vi "Actor Core.vi"(8 "error in":errorcluster, 11 "AE75TX in":refnum<class "AE75TX.lvclass">) -> (0 "error out":errorcluster, 3 "Actor out":refnum<class "Actor.lvclass">)   [LabVIEW 2018, in "AE75TX Actor.lvlib" / "AE75TX.lvclass"]
doc: "(<B>Filename</B>: Actor Framework.lvlib:Actor.lvclass:Actor Core.vi)\n\nReceives messages to the actor, reacts to them, and initiates any error handling that may shut the actor down.\n\nDescendant classes may override this VI to append parallel tasks for the actor to complete while it handles messages. Overrides use the Call Parent Method node."
uses:
  AE75TX.lvclass
  C:/Program Files (x86)/National Instruments/LabVIEW 2018/vi.lib/ActorFramework/Actor/Actor.lvclass
  <vilib>/ActorFramework/Actor/Actor.lvclass
  Controls/DDS State.ctl
  Controls/Modbus State.ctl
  AE75TX.lvclass/AE75TX.ctl
  <vilib>/ActorFramework/Actor/Actor.lvclass/Actor.ctl
  <vilib>/ActorFramework/Message Enqueuer/Message Enqueuer.lvclass/Message Enqueuer.ctl
  <vilib>/ORNL/CSEISMIC DDS/CSEISMIC DDS Base/CSEISMIC DDS.lvclass/CSEISMIC DDS.ctl
  <vilib>/ORNL/CSEISMIC DDS/DDS Writer/DDS Writer.lvclass
  C:/Program Files (x86)/National Instruments/LabVIEW 2018/vi.lib/ORNL/CSEISMIC DDS/CSEISMIC DDS Base/CSEISMIC DDS.lvclass
  <vilib>/ORNL/CSEISMIC DDS/DDS Reader/DDS Reader.lvclass
  <extravilib>/ChannelInstances/Stream-u16/EndpointRead.vi
  <vilib>/ActorFramework/Message Enqueuer/Init from Existing Queue.vi
  <vilib>/ActorFramework/Message Enqueuer/Enqueue.vi
  <vilib>/ORNL/CSEISMIC DDS/CSEISMIC DDS Base/Accessors/Write DDS Reference.vi
  <vilib>/ORNL/CSEISMIC DDS/CSEISMIC DDS Base/Accessors/Read DDS Reference.vi
  <extravilib>/ChannelInstances/Stream-u16/Endpoint.vi
  <vilib>/ActorFramework/Stop Msg/Stop Msg.lvclass
  C:/Program Files (x86)/National Instruments/LabVIEW 2018/vi.lib/ActorFramework/Message/Message.lvclass
  <extravilib>/ChannelInstances/Tag-t'CSEISMIC DDS.lvlib-CSEISMIC DDS.lvclass-IED_Status.ctl'/Instantiate.vi
  <extravilib>/ChannelInstances/Tag-t'CSEISMIC DDS.lvlib-CSEISMIC DDS.lvclass-DER_Status.ctl'/Instantiate.vi
  <extravilib>/ChannelInstances/Tag-t'CSEISMIC DDS.lvlib-CSEISMIC DDS.lvclass-DER_Measurement.ctl'/Instantiate.vi
  <extravilib>/ChannelInstances/Stream-u16/Instantiate.vi
  <vilib>/Modbus/master/Create Master Instance (TCP).vi
  <extravilib>/ChannelInstances/Tag-t'CSEISMIC DDS.lvlib-CSEISMIC DDS.lvclass-IED_Status.ctl'/Endpoint.vi
  <extravilib>/ChannelInstances/Tag-t'CSEISMIC DDS.lvlib-CSEISMIC DDS.lvclass-DER_Status.ctl'/Endpoint.vi
  <extravilib>/ChannelInstances/Tag-t'CSEISMIC DDS.lvlib-CSEISMIC DDS.lvclass-DER_Measurement.ctl'/Endpoint.vi
  <extravilib>/ChannelInstances/Stream-u16/)Channel.vi
  <resource>/ChannelSupport/_ChannelSupport/WaitIfNeeded.vi
  <vilib>/ActorFramework/Message Priority Queue/Priority Enqueue.vi
  <vilib>/ORNL/CSEISMIC DDS/CSEISMIC DDS Base/Error Handler.vi
  <extravilib>/ChannelInstances/Tag-t'CSEISMIC DDS.lvlib-CSEISMIC DDS.lvclass-IED_Status.ctl'/EndpointRead.vi
  <extravilib>/ChannelInstances/Tag-t'CSEISMIC DDS.lvlib-CSEISMIC DDS.lvclass-DER_Status.ctl'/EndpointRead.vi
  <extravilib>/ChannelInstances/Tag-t'CSEISMIC DDS.lvlib-CSEISMIC DDS.lvclass-DER_Measurement.ctl'/EndpointRead.vi
  <vilib>/Modbus/master/Modbus Master.lvclass
  <vilib>/ActorFramework/Message Enqueuer/Message Enqueuer.lvclass
  <vilib>/RTI DDS Toolkit/Library/LVDDS_library.lvlib
  <extravilib>/ChannelInstances/Tag-t'CSEISMIC DDS.lvlib-CSEISMIC DDS.lvclass-IED_Status.ctl'.lvlib
  <extravilib>/ChannelInstances/Tag-t'CSEISMIC DDS.lvlib-CSEISMIC DDS.lvclass-DER_Status.ctl'.lvlib
  <extravilib>/ChannelInstances/Tag-t'CSEISMIC DDS.lvlib-CSEISMIC DDS.lvclass-DER_Measurement.ctl'.lvlib
  <extravilib>/ChannelInstances/Stream-u16.lvlib
panel:
  out "MicrogridID":u8
  out "DDS State":T1
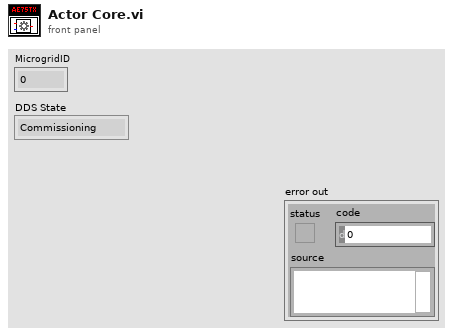
[diagram p1: front panel]
types:
  T1 = typedef "AE75TX Actor.lvlib/AE75TX.lvclass/DDS State.ctl" = enum16{"Commissioning", "CheckID", "InitDDS", "ReadDDS", "WriteDDS", "CheckClose", "Close", "Shutdown"}
  T2 = typedef "AE75TX Actor.lvlib/AE75TX.lvclass/Modbus State.ctl" = enum16{"Initialize", "Read", "Write", "Close"}
  T3 = typedef "AE75TX Actor.lvlib/AE75TX.lvclass/Scaling Coefficients Measurements.ctl" = cluster{"Current":dbl, "Voltage":dbl, "Real Power":dbl, "Reactive Power":dbl, "Frequency":dbl}
  T4 = typedef "AE75TX Actor.lvlib/AE75TX.lvclass/Modbus Configuration Cluster.ctl" = cluster{"IP Address":string, "Port":u16, "DeviceID":T5}
  T5 = typedef "CSEISMIC DDS.lvlib/CSEISMIC DDS.lvclass/DeviceID.ctl" = string
  T6 = typedef "CSEISMIC DDS.lvlib/CSEISMIC DDS.lvclass/DER_Info.ctl" = cluster{"DeviceID":T5, "LineConfig":u8[], "NominalVoltage(V)":dbl, "PowerRating(kVA)":dbl, "VFControl":bool, "PControl":bool, "QControl":bool, "PFControl":bool, "PVControl":bool, "Droop":bool, "DroopConfigurable":bool, "Unbalanced":bool}
  T7 = typedef "CSEISMIC DDS.lvlib/CSEISMIC DDS.lvclass/DER_Measurement.ctl" = cluster{"DeviceID":T5, "Voltage":dbl[], "Current":dbl[], "RealPower":dbl[], "ReactivePower":dbl[], "LineConfig":u8[], "Frequency":dbl}
  T8 = typedef "CSEISMIC DDS.lvlib/CSEISMIC DDS.lvclass/DER_Status.ctl" = cluster{"DeviceID":T5, "VFControl":bool, "PControl":bool, "QControl":bool, "PFControl":bool, "PVControl":bool, "Droop":bool, "Unbalanced":bool, "MicrogridVF":bool, "RealDroop(kW)":T9, "ReactiveDroop(kVar)":T9}
  T9 = typedef "CSEISMIC DDS.lvlib/CSEISMIC DDS.lvclass/DroopCurve.ctl" = cluster{"XMin":dbl, "XMax":dbl, "YMin":dbl, "YMax":dbl}
  T10 = typedef "CSEISMIC DDS.lvlib/CSEISMIC DDS.lvclass/IED_Status.ctl" = cluster{"DeviceID":T5, "Timestamp":T11, "MicrogridID":u8, "Active":bool, "Inactive":bool, "Error":i32, "Fault":bool, "ErrorString":string}
  T11 = typedef "CSEISMIC DDS.lvlib/CSEISMIC DDS.lvclass/Timestamp.ctl" = cluster{"Seconds":u64, "Remainder":u64}
  T12 = typedef "Tag-t'CSEISMIC DDS.lvlib-CSEISMIC DDS.lvclass-DER_Status.ctl'.lvlib/))Channel.ctl" = refnum<queue>
  T13 = typedef "Tag-t'CSEISMIC DDS.lvlib-CSEISMIC DDS.lvclass-DER_Measurement.ctl'.lvlib/))Channel.ctl" = refnum<queue>
  T14 = typedef "Tag-t'CSEISMIC DDS.lvlib-CSEISMIC DDS.lvclass-IED_Status.ctl'.lvlib/))Channel.ctl" = refnum<queue>
  T15 = typedef "CSEISMIC DDS.lvlib/CSEISMIC DDS.lvclass/IED_setMicrogridID.ctl" = cluster{"DeviceID":T5, "MicrogridID":u8}
  T16 = typedef "LVDDS_library.lvlib/DDS Sample Info.ctl" = cluster{"DDS_SampleStateKind":enum32{"DDS_INVALID_SAMPLE_STATE", "DDS_READ_SAMPLE_STATE", "DDS_NOT_READ_SAMPLE_STATE"}, "DDS_ViewStateKind":enum32{"DDS_INVALID_SAMPLE_STATE", "DDS_NEW_VIEW_STATE", "DDS_NOT_NEW_VIEW_STATE"}, "DDS_InstanceStateKind":enum32{"DDS_INVALID_STATE", "DDS_ALIVE_INSTANCE_STATE", "DDS_NOT_ALIVE_DISPOSED_INSTANCE_STATE", "", "DDS_NOT_ALIVE_NO_WRITERS_INSTANCE_STATE"}, "sec":i32, "nanosec":u32, "valid_data":bool}
  T17 = typedef "CSEISMIC DDS.lvlib/CSEISMIC DDS.lvclass/DER_SetPointP.ctl" = cluster{"DeviceID":T5, "RealPower (kW)":dbl[]}
  T18 = typedef "Stream-u16.lvlib/)Channel.ctl" = refnum<queue>
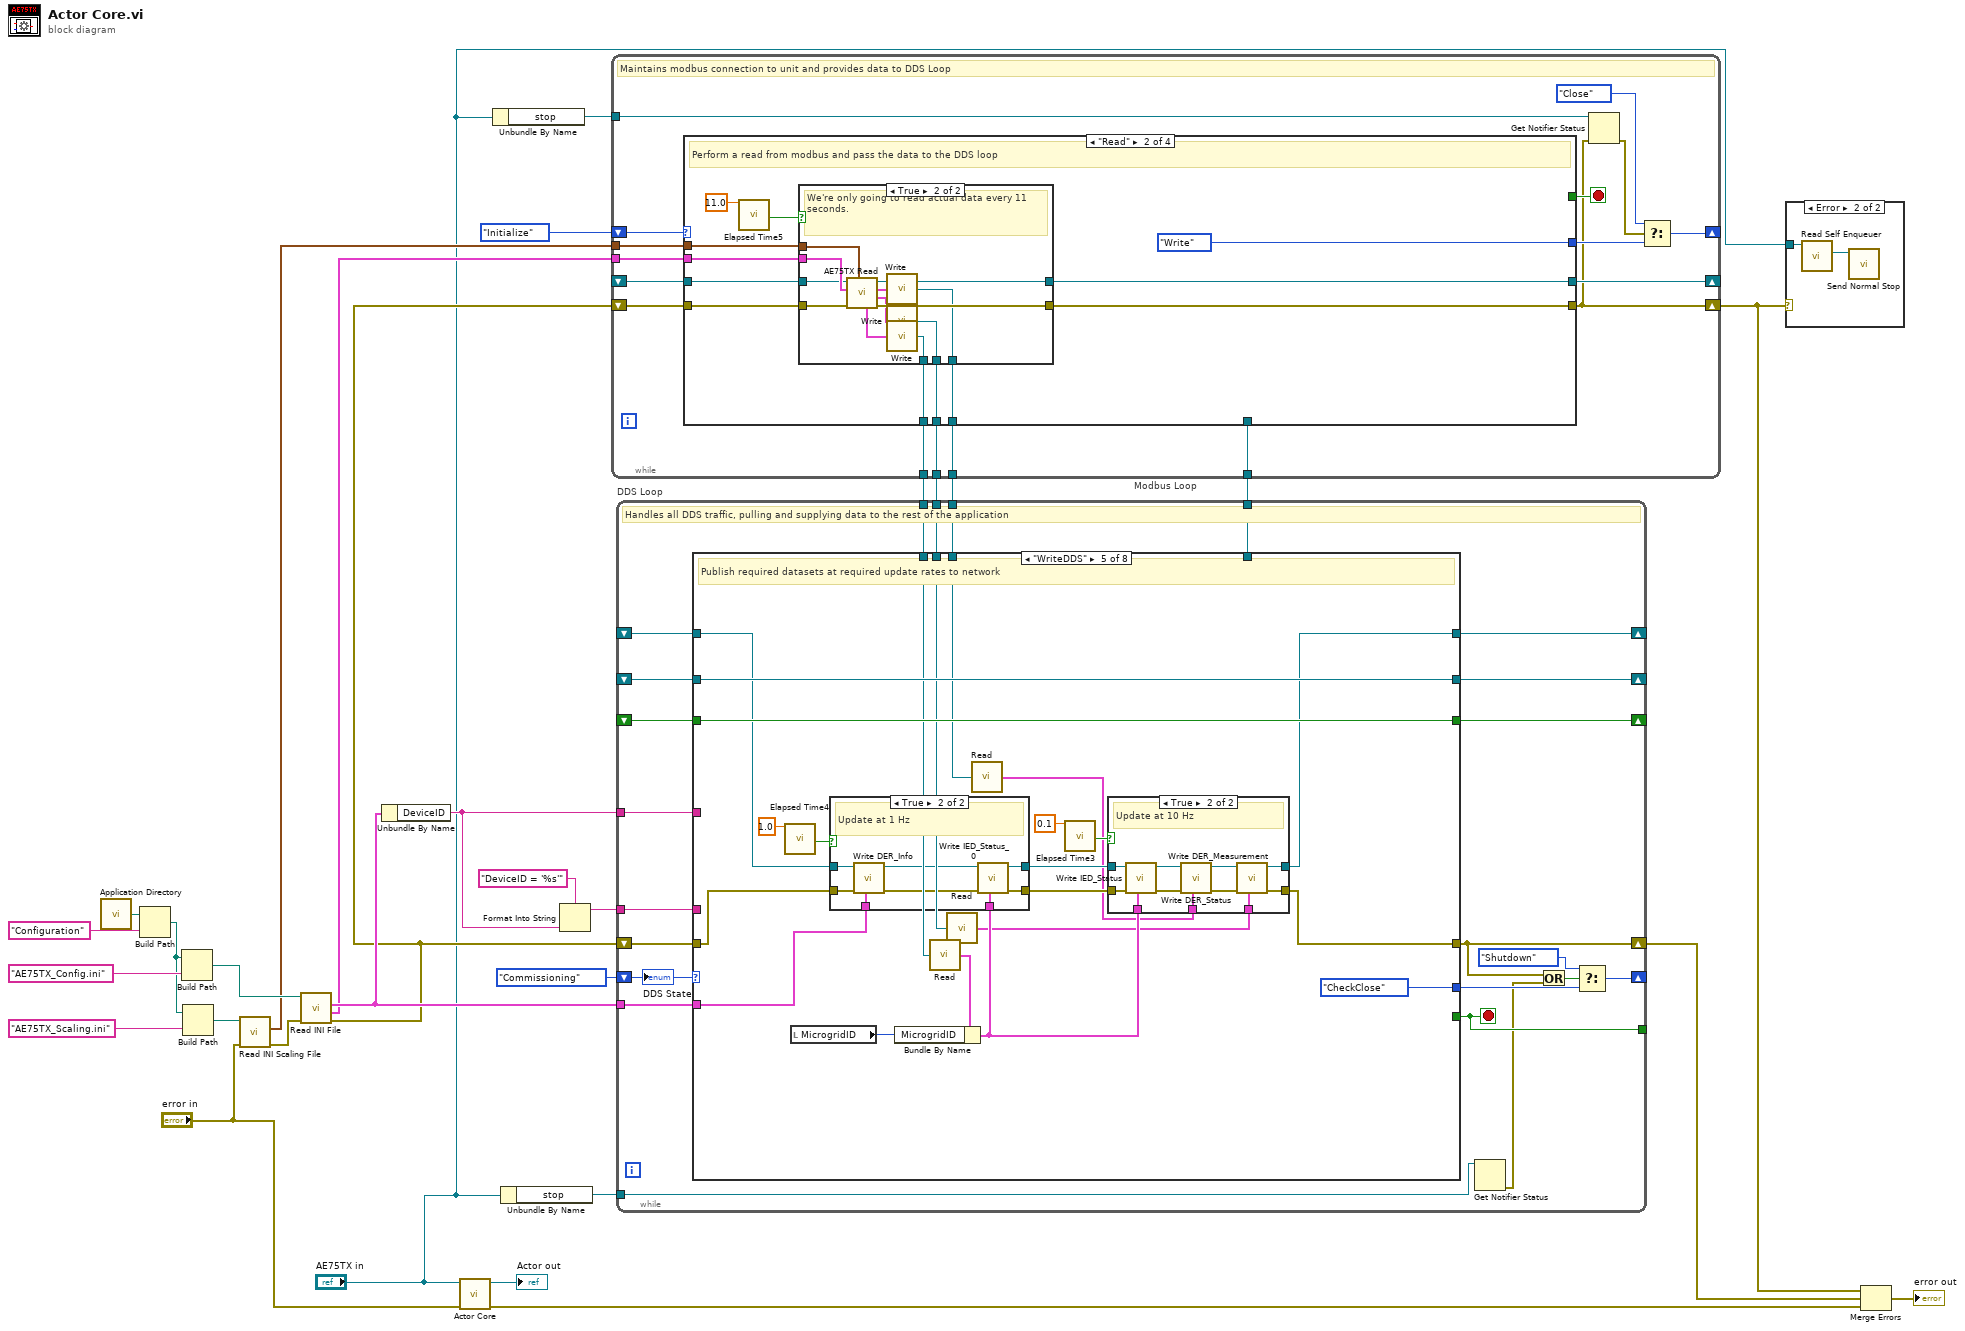
[diagram p0: block diagram]
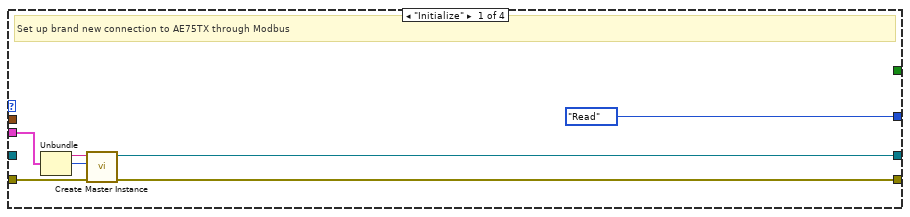
[diagram p3: hidden frame]
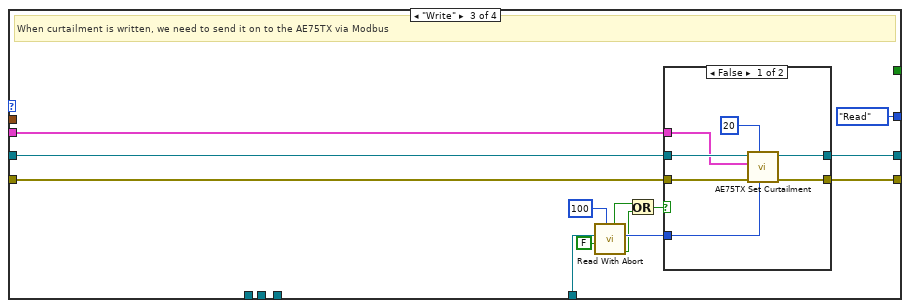
[diagram p5: hidden frame]
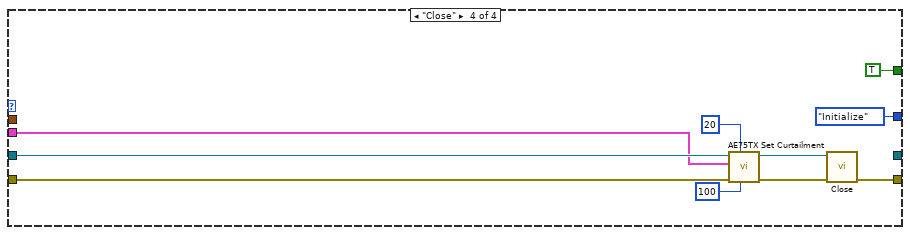
[diagram p7: hidden frame]
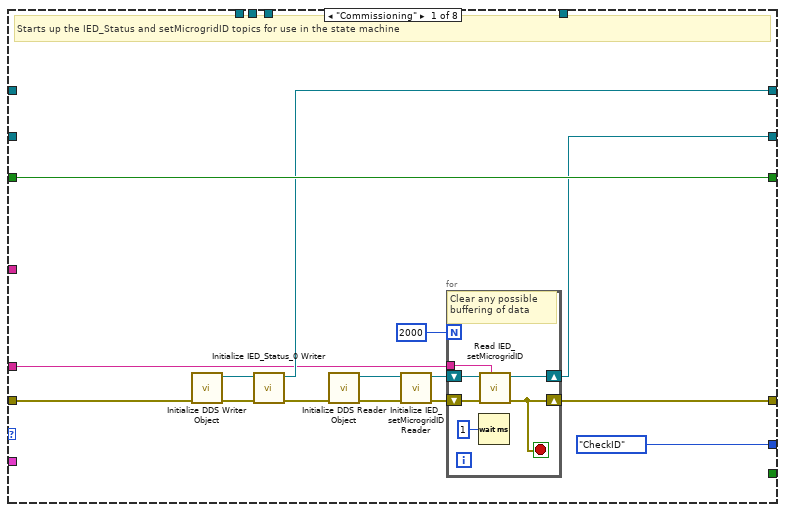
[diagram p8: hidden frame]
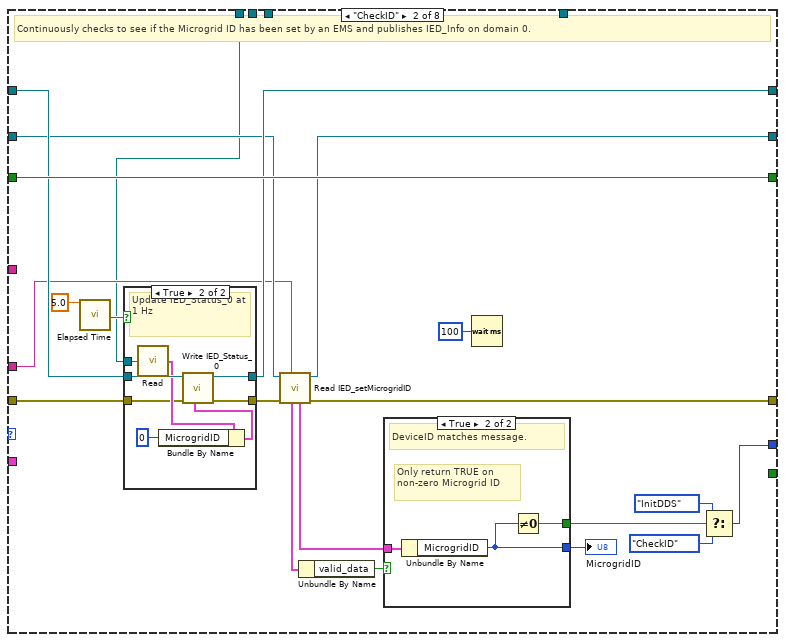
[diagram p9: hidden frame]
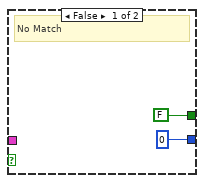
[diagram p11: hidden frame]
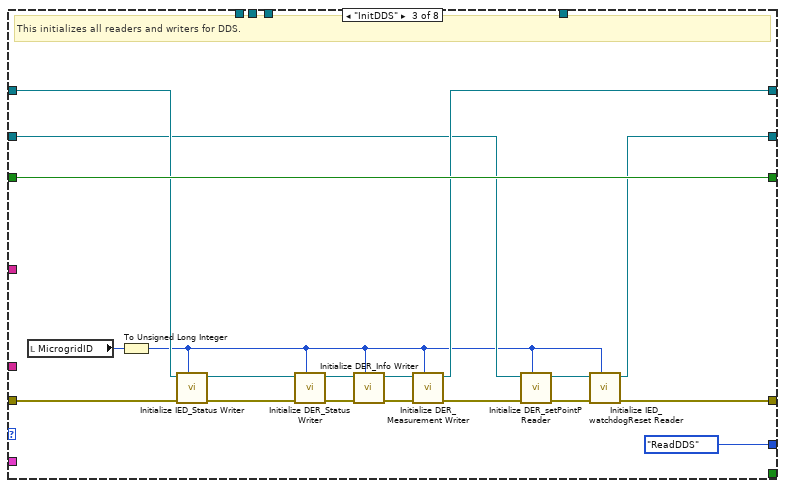
[diagram p12: hidden frame]
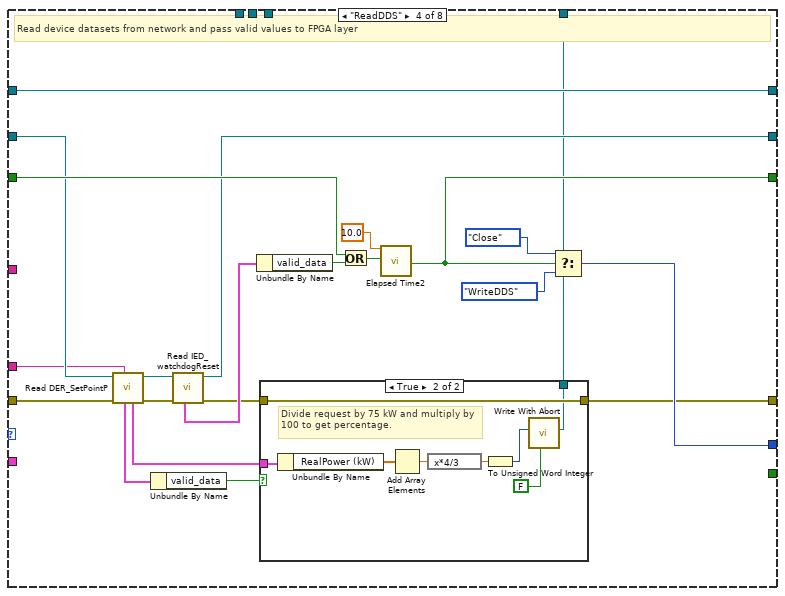
[diagram p13: hidden frame]
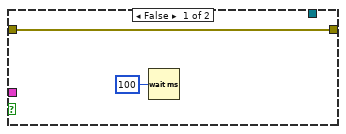
[diagram p14: hidden frame]
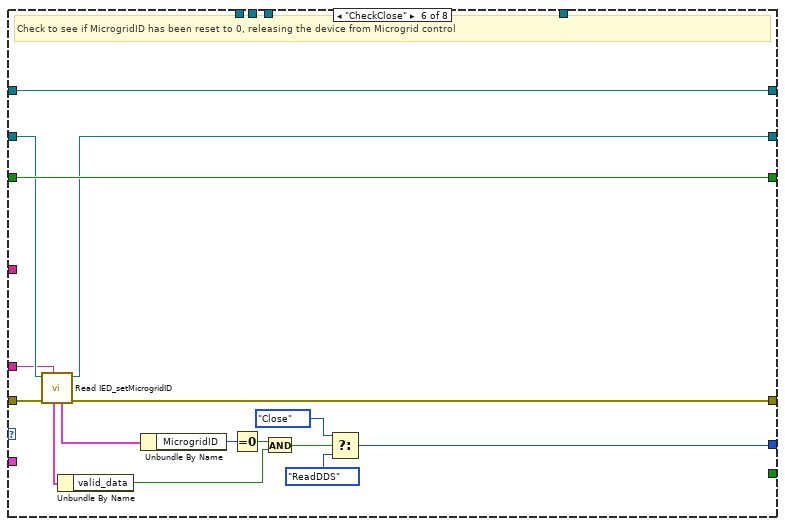
[diagram p17: hidden frame]
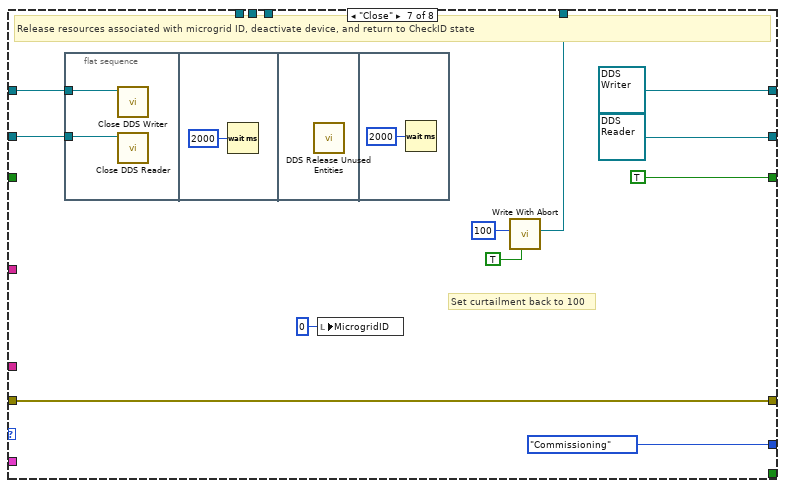
[diagram p18: hidden frame]
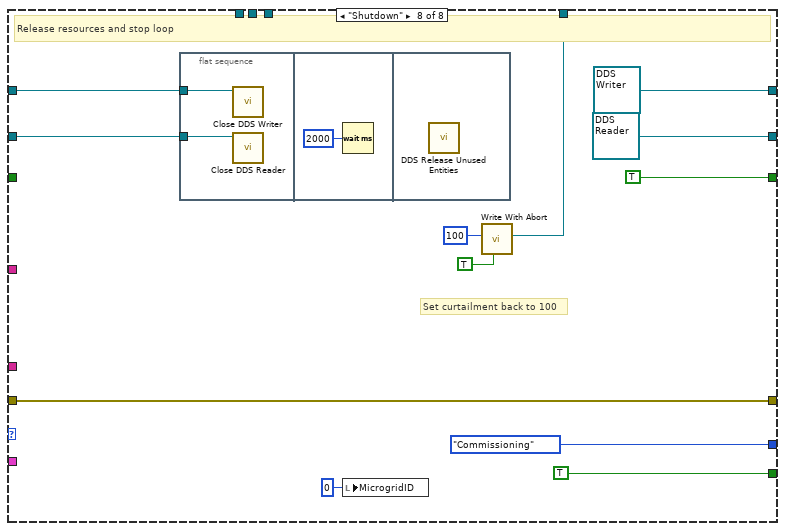
[diagram p19: hidden frame]
diagram:
  n1 = call <vilib>:"Application Directory.vi"() -> ("Application Directory"=w25:path)
  n2 = Build Path(base path=w25, name or relative path="Configuration") -> (appended path=w17:path)
  n3 = Build Path(base path=w17, name or relative path="AE75TX_Config.ini") -> (appended path=w20:path)
  n4 = Build Path(base path=w17, name or relative path="AE75TX_Scaling.ini") -> (appended path=w16:path)
  n5 = call "Read INI Scaling File.vi"("error in"="error in", "Path"=w16) -> ("error out"=w19:errorcluster, "Scaling Coefficients"=w7:T3)  [unwired: 8 in]
  n6 = call "Read INI File.vi"("error in"=w19, "Path"=w20) -> ("error out"=w8:errorcluster, "Modbus Configuration"=w9:T4, "DER_Info"=w12:T6)  [unwired: 7 in]
  n7 = Unbundle By Name(w12) -> ("DeviceID"=w23:T5)
  n8 = call-parent "Actor Core.vi"("error in"="error in", "Actor in"="AE75TX in") -> ("error out"=w30:errorcluster, "Actor out"=→"Actor out":refnum<class "Actor.lvclass">)  [unwired: 8 in]
  n9 = Unbundle By Name("AE75TX in") -> ("stop"=w11:refnum<notifier>)
  n10 = Unbundle By Name("AE75TX in") -> ("stop"=w14:refnum<notifier>)
  n11 = Format Into String(format string="DeviceID = '%s'" ("Query condition"), w23) -> (resulting string=w22:string)  [unwired: 2 in, 1 out]
  n12 = while "Modbus Loop" {
    tunnel: w11 -> [w47]
    shift-right: [w33] -> _
    shift-left: Modbus_State."Initialize" -> [w46]
    tunnel: w9 -> [w45]
    shift-right: [w44] -> _
    shift-left: _ -> [w42]
    shift-right: [w31] -> w1
    shift-left: w8 -> [w43]
    tunnel: w7 -> [w41]
    tunnel: w6 -> [w40]
    tunnel: [w39] -> w5
    tunnel: [w38] -> w4
    tunnel: [w37] -> w3
    stop <- w36 stop-if-true
    # "Maintains modbus connection to unit and provides data to DDS Loop"
    n13 = case shown="\"Read\"" w46 {
      tunnel: w45 -> [w52 w66 w87 w104]
      tunnel: [w51 w63 w85 _] -> w44
      tunnel: w43 -> [w50 w64 w92 w106]
      tunnel: [w49 w62 w84 w112] -> w31
      tunnel: [Modbus_State."Read" Modbus_State."Write" Modbus_State."Read" Modbus_State."Initialize"] -> w34
      tunnel: w42 -> [_ w65 w93 w107]
      tunnel: w41 -> [_ w58 _ _]
      tunnel: w40 -> [_ _ w91 _]
      tunnel: [_ w57 _ _] -> w39
      tunnel: [_ w56 _ _] -> w38
      tunnel: [_ w55 _ _] -> w37
      tunnel: [_ _ _ TRUE] -> w36
      frame "Initialize" {
        # "Set up brand new connection to AE75TX through Modbus"
        n14 = Unbundle(w52) -> ("IP Address"=w53:string, "Port"=w54:u16)  [unwired: 1 out]
        n15 = call-poly <vilib>:"Create Master Instance.vi"("error in (no error)"=w50, "port (502)"=w54, "address"=w53) -> ("error out"=w49:errorcluster, "TCP master instance"=w51:refnum<class "Modbus Master.lvclass">)  [unwired: 7 in]
      }
      frame "Read" {
        # "Perform a read from modbus and pass the data to the DDS loop"
        n16 = call "Elapsed Time5"("Time Target (s)"=11.0) -> ("Time has Elapsed"=w60:bool)  [unwired: 11 in, 7 out]
        n17 = case shown="True" w60 {
          tunnel: w66 -> [_ w80]
          tunnel: w65 -> [w67 w79]
          tunnel: w64 -> [w68 w78]
          tunnel: [w67 w77] -> w63
          tunnel: [w68 w76] -> w62
          tunnel: w58 -> [_ w75]
          tunnel: [_ w72] -> w57
          tunnel: [_ w71] -> w56
          tunnel: [_ w70] -> w55
          frame False {
            # "Do nothing"
          }
          frame True {
            # "We're only going to read actual data every 11 seconds."
            n18 = call "AE75TX Read.vi"("Scaling Coefficients"=w75, "error in"=w78, "Modbus Configuration"=w80, "Modbus Master in"=w79) -> ("error out"=w76:errorcluster, "DER_Measurement"=w73:T7, "DER_Status"=w74:T8, "Modbus Master out"=w77:refnum<class "Modbus Master.lvclass">, "IED_Status"=w69:T10)  [unwired: 3 in]
            n19 = call <extravilib>:"Write.vi"("element"=w74) -> ("channel"=w71:T12)  [unwired: 1 out]
            n20 = call <extravilib>:"Write.vi"("element"=w73) -> ("channel"=w72:T13)  [unwired: 1 out]
            n21 = call <extravilib>:"Write.vi"("element"=w69) -> ("channel"=w70:T14)  [unwired: 1 out]
          }
        }
      }
      frame "Write" {
        # "When curtailment is written, we need to send it on to the AE75TX via Modbus"
        n22 = call <extravilib>:"Read With Abort.vi"("timeout in ms (-1)"=100, "abort"=FALSE, "channel"=w91) -> ("element"=w90:u16, "aborted?"=w81:bool, "timed out?"=w88:bool)  [unwired: 3 in, 3 out]
        n23 = Or(x=w88, y=w81) -> (x .or. y?=w82:bool)
        n24 = case shown="False" w82 {
          tunnel: w93 -> [w99 w102]
          tunnel: w92 -> [w98 w101]
          tunnel: w90 -> [w94 _]
          tunnel: [w97 w102] -> w85
          tunnel: [w96 w101] -> w84
          tunnel: w87 -> [w95 _]
          frame False {
            n25 = call "AE75TX Set Curtailment.vi"("Curtailment (%)"=w94, "Ramp Rate (kVA/s)"=u16 20, "error in"=w98, "Modbus Configuration"=w95, "Modbus Master in"=w99) -> ("error out"=w96:errorcluster, "Modbus Master out"=w97:refnum<class "Modbus Master.lvclass">)  [unwired: 5 in]
          }
          frame True {
          }
        }
      }
      frame "Close" {
        n26 = call "AE75TX Set Curtailment.vi"("Curtailment (%)"=u16 100, "Ramp Rate (kVA/s)"=u16 20, "error in"=w106, "Modbus Configuration"=w104, "Modbus Master in"=w107) -> ("error out"=w108:errorcluster, "Modbus Master out"=w109:refnum<class "Modbus Master.lvclass">)  [unwired: 5 in]
        n27 = call-dynamic "Close.vi"("error in (no error)"=w108, "Modbus master in"=w109) -> ("error out"=w112:errorcluster)  [unwired: 9 in]
      }
    }
    n28 = Get Notifier Status(notifier=w47, error in (no error)=w31) -> (error out=w35:errorcluster)  [unwired: 4 out]
    n29 = Select(t=Modbus_State."Close", s=w35, f=w34) -> (s? t:f=w33:T2)
  }
  n30 = while "DDS Loop" {
    shift-right: [w133] -> _
    shift-left: DDS_State."Commissioning" -> [w135]
    tunnel: w23 -> [w134]
    shift-right: [w121] -> w13
    shift-left: w8 -> [w117]
    shift-right: [w122] -> _
    shift-left: _ -> [w129]
    tunnel: [w128] -> _
    tunnel: w22 -> [w123]
    shift-right: [w125] -> _
    shift-left: _ -> [w127]
    shift-right: [w124] -> _
    shift-left: _ -> [w126]
    tunnel: w12 -> [w120]
    tunnel: w14 -> [w119]
    tunnel: [w116] -> w6
    tunnel: w5 -> [w114]
    tunnel: w4 -> [w113]
    tunnel: w3 -> [w115]
    stop <- w128 stop-if-true
    # "Handles all DDS traffic, pulling and supplying data to the rest of the application"
    n31 = case shown="\"CheckID\"" w135 {
      tunnel: [DDS_State."CheckID" w173 DDS_State."ReadDDS" w231 DDS_State."CheckClose" w301 DDS_State."Commissioning" ("f") DDS_State."Commissioning" ("f")] -> w132
      tunnel: [w149 w166 w206 w220 w262 w297 w314 w323] -> w121
      tunnel: w134 -> [_ _ _ _ _ _ _ _]
      tunnel: w117 -> [w136 w157 w208 w218 w244 w298 w314 w323]
      tunnel: [_ _ _ _ _ _ _ TRUE] -> w128
      tunnel: [w148 w169 w209 w228 w257 w300 TRUE ("Time has Elapsed") TRUE ("Time has Elapsed")] -> w122
      tunnel: w129 -> [w148 w169 w209 w227 w257 w300 _ _]
      tunnel: w127 -> [_ w168 w205 w226 w255 w293 w311 w325]
      tunnel: w126 -> [_ w164 w197 w219 w256 w299 w310 w324]
      tunnel: [w146 w167 w203 w226 w254 w293 refnum<class "DDS Writer.lvclass"> refnum ("DDS Writer out") refnum<class "DDS Writer.lvclass"> refnum ("DDS Writer out")] -> w125
      tunnel: [w145 w163 w202 w222 w256 w294 refnum<class "DDS Reader.lvclass"> refnum ("DDS Reader out") refnum<class "DDS Reader.lvclass"> refnum ("DDS Reader out")] -> w124
      tunnel: w123 -> [w138 w161 _ w213 _ w295 _ _]
      tunnel: w120 -> [_ _ _ _ w253 _ _ _]
      tunnel: [_ _ _ w212 _ _ w307 w320] -> w116
      tunnel: w115 -> [_ w158 _ _ w250 _ _ _]
      tunnel: w114 -> [_ _ _ _ w249 _ _ _]
      tunnel: w113 -> [_ _ _ _ w248 _ _ _]
      frame "Commissioning" {
        # "Starts up the IED_Status and setMicrogridID topics for use in the state machine"
        n32 = call <vilib>:"Initialize DDS Writer Object.vi"("error in"=w136) -> ("error out"=w143:errorcluster, "DDS Writer out"=w142:refnum<class "DDS Writer.lvclass">)  [unwired: 9 in]
        n33 = call <vilib>:"Initialize IED_Status_0 Writer.vi"("error in"=w143, "DDS Writer in"=w142) -> ("error out"=w141:errorcluster, "DDS Writer out"=w146:refnum<class "DDS Writer.lvclass">)  [unwired: 8 in]
        n34 = call <vilib>:"Initialize DDS Reader Object.vi"("error in"=w141) -> ("error out"=w140:errorcluster, "DDS Reader out"=w139:refnum<class "DDS Reader.lvclass">)  [unwired: 9 in]
        n35 = call <vilib>:"Initialize IED_setMicrogridID Reader.vi"("error in"=w140, "DDS Reader in"=w139) -> ("error out"=w144:errorcluster, "DDS Reader out"=w147:refnum<class "DDS Reader.lvclass">)  [unwired: 8 in]
        n36 = for {
          N: 2000 -> [_]
          shift-right: [w154] -> w145
          shift-left: w147 -> [w155]
          shift-right: [w152] -> w149
          shift-left: w144 -> [w153]
          tunnel: w138 -> [w151]
          stop <- w152 stop-if-true
          # "Clear any possible buffering of data"
          n37 = Wait (ms)(milliseconds to wait=u32 1) -> ()  [unwired: 1 out]
          n38 = call <vilib>:"Read IED_setMicrogridID.vi"("Query condition"=w151, "error in"=w153, "DDS Reader in"=w155) -> ("error out"=w152:errorcluster, "DDS Reader out"=w154:refnum<class "DDS Reader.lvclass">)  [unwired: 5 in, 2 out]
        }
      }
      frame "CheckID" {
        # "Continuously checks to see if the Microgrid ID has been set by an EMS and publishes IED_Info on domain 0."
        n39 = call "Elapsed Time"("Time Target (s)"=5.0) -> ("Time has Elapsed"=w171:bool)  [unwired: 11 in, 7 out]
        n40 = case shown="True" w171 {
          tunnel: [w178 w186] -> w165
          tunnel: w168 -> [w179 w187]
          tunnel: [w179 w185] -> w167
          tunnel: w158 -> [_ w183]
          tunnel: w157 -> [w178 w180]
          frame False {
          }
          frame True {
            # "Update IED_Status_0 at 1 Hz"
            n41 = call <extravilib>:"Read.vi"("channel"=w183) -> ("element"=w182:T10)  [unwired: 1 in, 1 out]
            n42 = Bundle By Name(cluster=w182, "MicrogridID"=u8 0) -> (w181:T10)
            n43 = call <vilib>:"Write IED_Status_0.vi"("IED_Status"=w181, "error in"=w180, "DDS Writer in"=w187) -> ("error out"=w186:errorcluster, "DDS Writer out"=w185:refnum<class "DDS Writer.lvclass">)  [unwired: 7 in]
          }
        }
        n44 = call <vilib>:"Read IED_setMicrogridID.vi"("Query condition"=w161, "error in"=w165, "DDS Reader in"=w164) -> ("error out"=w166:errorcluster, "DDS Reader out"=w163:refnum<class "DDS Reader.lvclass">, "data"=w162:T15, "DDS Sample Info"=w160:T16)  [unwired: 5 in]
        n45 = Unbundle By Name(w160) -> ("valid_data"=w159:bool)
        n46 = case shown="True" w159 {
          tunnel: w162 -> [_ w192]
          tunnel: [u8 0 ("MicrogridID") w191] -> w172
          tunnel: [FALSE w190] -> w176
          frame False {
            # "No Match"
          }
          frame True {
            # "Only return TRUE on non-zero Microgrid ID"
            # "DeviceID matches message."
            n47 = Unbundle By Name(w192) -> ("MicrogridID"=w191:u8)
            n48 = Not Equal To 0?(x=w191) -> (x != 0?=w190:bool)
          }
        }
        "MicrogridID" <- w172
        n49 = Wait (ms)(milliseconds to wait=u32 100) -> ()  [unwired: 1 out]
        n50 = Select(t=DDS_State."InitDDS", s=w176, f=DDS_State."CheckID") -> (s? t:f=w173:T1)
      }
      frame "InitDDS" {
        # "This initializes all readers and writers for DDS."
        n51 = local read "MicrogridID"() -> (w210:u8)
        n52 = To Unsigned Long Integer(number=w210) -> (unsigned 32bit integer=w193:u32)
        n53 = call <vilib>:"Initialize IED_Status Writer.vi"("MicrogridID"=w193, "error in"=w208, "DDS Writer in"=w205) -> ("error out"=w200:errorcluster, "DDS Writer out"=w201:refnum<class "DDS Writer.lvclass">)  [unwired: 7 in]
        n54 = call <vilib>:"Initialize DER_Status Writer.vi"("MicrogridID"=w193, "error in"=w200, "DDS Writer in"=w201) -> ("error out"=w199:errorcluster, "DDS Writer out"=w198:refnum<class "DDS Writer.lvclass">)  [unwired: 7 in]
        n55 = call <vilib>:"Initialize DER_Info Writer.vi"("MicrogridID"=w193, "error in"=w199, "DDS Writer in"=w198) -> ("error out"=w207:errorcluster, "DDS Writer out"=w204:refnum<class "DDS Writer.lvclass">)  [unwired: 7 in]
        n56 = call <vilib>:"Initialize DER_Measurement Writer.vi"("MicrogridID"=w193, "error in"=w207, "DDS Writer in"=w204) -> ("error out"=w196:errorcluster, "DDS Writer"=w203:refnum<class "DDS Writer.lvclass">)  [unwired: 7 in]
        n57 = call <vilib>:"Initialize DER_setPointP Reader.vi"("MicrogridID"=w193, "error in"=w196, "DDS Reader in"=w197) -> ("error out"=w194:errorcluster, "DDS Reader out"=w195:refnum<class "DDS Reader.lvclass">)  [unwired: 7 in]
        n58 = call <vilib>:"Initialize IED_watchdogReset Reader.vi"("MicrogridID"=w193, "error in"=w194, "DDS Reader in"=w195) -> ("error out"=w206:errorcluster, "DDS Reader out"=w202:refnum<class "DDS Reader.lvclass">)  [unwired: 7 in]
      }
      frame "ReadDDS" {
        # "Read device datasets from network and pass valid values to FPGA layer"
        n59 = call <vilib>:"Read DER_SetPointP.vi"("Query condition"=w213, "error in"=w218, "DDS Reader in"=w219) -> ("error out"=w216:errorcluster, "DDS Reader out"=w217:refnum<class "DDS Reader.lvclass">, "data"=w214:T17, "DDS Sample Info"=w215:T16)  [unwired: 5 in]
        n60 = Unbundle By Name(w215) -> ("valid_data"=w223:bool)
        n61 = call <vilib>:"Read IED_watchdogReset.vi"("error in"=w216, "DDS Reader in"=w217) -> ("error out"=w221:errorcluster, "DDS Reader out"=w222:refnum<class "DDS Reader.lvclass">, "DDS Sample Info"=w225:T16)  [unwired: 6 in, 1 out]
        n62 = Unbundle By Name(w225) -> ("valid_data"=w224:bool)
        n63 = case shown="True" w223 {
          tunnel: w221 -> [w235 w238]
          tunnel: [w235 w238] -> w220
          tunnel: w214 -> [_ w243]
          tunnel: [_ w237] -> w212
          frame False {
            n64 = Wait (ms)(milliseconds to wait=u32 100) -> ()  [unwired: 1 out]
          }
          frame True {
            # "Divide request by 75 kW and multiply by 100 to get percentage."
            n65 = Unbundle By Name(w243) -> ("RealPower (kW)"=w242:dbl[])
            n66 = Add Array Elements(numeric array=w242) -> (sum=w241:dbl)
            n67 = expression code="x*4/3"(w241) -> (w240:dbl)
            n68 = To Unsigned Word Integer(number=w240) -> (unsigned 16bit integer=w239:u16)
            n69 = call <extravilib>:"Write With Abort.vi"("abort"=FALSE, "element"=w239) -> ("channel"=w237:T18)  [unwired: 6 in, 3 out]
          }
        }
        n70 = Or(x=w227, y=w224) -> (x .or. y?=w229:bool)
        n71 = call "Elapsed Time2"("Time Target (s)"=10.0, "Reset"=w229) -> ("Time has Elapsed"=w228:bool)  [unwired: 10 in, 7 out]
        n72 = Select(t=DDS_State."Close", s=w228, f=DDS_State."WriteDDS") -> (s? t:f=w231:T1)
      }
      frame "WriteDDS" {
        # "Publish required datasets at required update rates to network"
        n73 = call "Elapsed Time4"("Time Target (s)"=1.0) -> ("Time has Elapsed"=w258:bool)  [unwired: 11 in, 7 out]
        n74 = local read "MicrogridID"() -> (w251:u8)
        n75 = call <extravilib>:"Read.vi"("channel"=w250) -> ("element"=w247:T10)  [unwired: 1 in, 1 out]
        n76 = Bundle By Name(cluster=w247, "MicrogridID"=w251) -> (w252:T10)
        n77 = case shown="True" w258 {
          tunnel: [w280 w287] -> w264
          tunnel: [w279 w288] -> w263
          tunnel: w253 -> [_ w286]
          tunnel: w255 -> [w280 w285]
          tunnel: w252 -> [_ w282]
          tunnel: w244 -> [w279 w281]
          frame False {
          }
          frame True {
            # "Update at 1 Hz"
            n78 = call <vilib>:"Write DER_Info.vi"("DER_Info"=w286, "error in"=w281, "DDS Writer in"=w285) -> ("error out"=w284:errorcluster, "DDS Writer out"=w283:refnum<class "DDS Writer.lvclass">)  [unwired: 7 in]
            n79 = call <vilib>:"Write IED_Status_0.vi"("IED_Status"=w282, "error in"=w284, "DDS Writer in"=w283) -> ("error out"=w288:errorcluster, "DDS Writer out"=w287:refnum<class "DDS Writer.lvclass">)  [unwired: 7 in]
          }
        }
        n80 = call <extravilib>:"Read.vi"("channel"=w249) -> ("element"=w245:T7)  [unwired: 1 in, 1 out]
        n81 = call <extravilib>:"Read.vi"("channel"=w248) -> ("element"=w246:T8)  [unwired: 1 in, 1 out]
        n82 = call "Elapsed Time3"("Time Target (s)"=0.1) -> ("Time has Elapsed"=w260:bool)  [unwired: 11 in, 7 out]
        n83 = case shown="True" w260 {
          tunnel: w264 -> [w267 w278]
          tunnel: w263 -> [w266 w277]
          tunnel: [w267 w276] -> w254
          tunnel: [w266 w275] -> w262
          tunnel: w252 -> [_ w268]
          tunnel: w246 -> [_ w270]
          tunnel: w245 -> [_ w269]
          frame False {
          }
          frame True {
            # "Update at 10 Hz"
            n84 = call <vilib>:"Write IED_Status.vi"("IED_Status"=w268, "error in"=w277, "DDS Writer in"=w278) -> ("error out"=w274:errorcluster, "DDS Writer out"=w273:refnum<class "DDS Writer.lvclass">)  [unwired: 7 in]
            n85 = call <vilib>:"Write DER_Status.vi"("DER_Status"=w270, "error in"=w274, "DDS Writer in"=w273) -> ("error out"=w272:errorcluster, "DDS Writer out"=w271:refnum<class "DDS Writer.lvclass">)  [unwired: 7 in]
            n86 = call <vilib>:"Write DER_Measurement.vi"("DER_Measurement"=w269, "error in"=w272, "DDS Writer in"=w271) -> ("error out"=w275:errorcluster, "DDS Writer out"=w276:refnum<class "DDS Writer.lvclass">)  [unwired: 7 in]
          }
        }
      }
      frame "CheckClose" {
        # "Check to see if MicrogridID has been reset to 0, releasing the device from Microgrid control"
        n87 = call <vilib>:"Read IED_setMicrogridID.vi"("Query condition"=w295, "error in"=w298, "DDS Reader in"=w299) -> ("error out"=w297:errorcluster, "DDS Reader out"=w294:refnum<class "DDS Reader.lvclass">, "data"=w296:T15, "DDS Sample Info"=w292:T16)  [unwired: 5 in]
        n88 = Unbundle By Name(w292) -> ("valid_data"=w291:bool)
        n89 = Unbundle By Name(w296) -> ("MicrogridID"=w304:u8)
        n90 = Equal To 0?(x=w304) -> (x = 0?=w290:bool)
        n91 = And(x=w290, y=w291) -> (x .and. y?=w289:bool)
        n92 = Select(t=DDS_State."Close", s=w289, f=DDS_State."ReadDDS") -> (s? t:f=w301:T1)
      }
      frame "Close" {
        # "Set curtailment back to 100"
        # "Release resources associated with microgrid ID, deactivate device, and return to CheckID state"
        n93 = flat-sequence {
          tunnel: w311 -> [w317]
          tunnel: w310 -> [w316]
          frame #0 {
            n94 = call <vilib>:"Close DDS Writer.vi"("DDS Writer in"=w317) -> ()  [unwired: 10 in, 1 out]
            n95 = call <vilib>:"Close DDS Reader.vi"("DDS Reader in"=w316) -> ()  [unwired: 10 in, 1 out]
          }
          frame #1 {
            n96 = Wait (ms)(milliseconds to wait=u32 2000) -> ()  [unwired: 1 out]
          }
          frame #2 {
            n97 = call <vilib>:"DDS Release Unused Entities.vi"() -> ()  [unwired: 10 in, 2 out]
          }
          frame #3 {
            n98 = Wait (ms)(milliseconds to wait=u32 2000) -> ()  [unwired: 1 out]
          }
        }
        n99 = local write "MicrogridID"(u8 0 ("MicrogridID")) -> ()
        n100 = call <extravilib>:"Write With Abort.vi"("abort"=TRUE, "element"=u16 100 ("Curtailment (%)")) -> ("channel"=w307:T18)  [unwired: 6 in, 3 out]
      }
      frame "Shutdown" {
        # "Set curtailment back to 100"
        # "Release resources and stop loop"
        n101 = flat-sequence {
          tunnel: w325 -> [w333]
          tunnel: w324 -> [w332]
          frame #0 {
            n102 = call <vilib>:"Close DDS Writer.vi"("DDS Writer in"=w333) -> ()  [unwired: 10 in, 1 out]
            n103 = call <vilib>:"Close DDS Reader.vi"("DDS Reader in"=w332) -> ()  [unwired: 10 in, 1 out]
          }
          frame #1 {
            n104 = Wait (ms)(milliseconds to wait=u32 2000) -> ()  [unwired: 1 out]
          }
          frame #2 {
            n105 = call <vilib>:"DDS Release Unused Entities.vi"() -> ()  [unwired: 10 in, 2 out]
          }
        }
        n106 = local write "MicrogridID"(u8 0 ("MicrogridID")) -> ()
        n107 = call <extravilib>:"Write With Abort.vi"("abort"=TRUE, "element"=u16 100 ("Curtailment (%)")) -> ("channel"=w320:T18)  [unwired: 6 in, 3 out]
      }
    }
    n108 = Get Notifier Status(notifier=w119) -> (error out=w118:errorcluster)  [unwired: 1 in, 4 out]
    n109 = Or(x=w121, y=w118) -> (x .or. y?=w130:bool)
    n110 = Select(t=DDS_State."Shutdown", s=w130, f=w132) -> (s? t:f=w133:T1)
    "DDS State" <- w135
  }
  n111 = case shown="Error" w1 {
    tunnel: "AE75TX in" -> [_ w336]
    frame No Error {
    }
    frame Error {
      n112 = call <vilib>:"Read Self Enqueuer.vi"("Actor"=w336) -> ("Self Enqueuer"=w335:refnum<class "Message Enqueuer.lvclass">)  [unwired: 10 in]
      n113 = call <vilib>:"Send Normal Stop.vi"("Message Enqueuer"=w335) -> ()  [unwired: 10 in, 1 out]
    }
  }
  n114 = Merge Errors(w1, w13, w30) -> (→"error out":errorcluster)
